vi "isForEditing.vi"(8 "error in (no error)":errorcluster, 11 "RampAction in":refnum<class "RampAction.lvclass">) -> (0 "error out":errorcluster, 2 "editing?":bool, 3 "RampAction out":refnum<class "RampAction.lvclass">)   [LabVIEW 2009, in "Views.lvlib" / "ScriptEditor.lvlib" / "RampAction.lvclass"]
uses:
  RampAction.lvclass
  Tools/Scripting/ScriptingEvent/ScriptEvents/Ramp/RampEvent/RampEvent.lvclass
  ActionPanel.lvclass
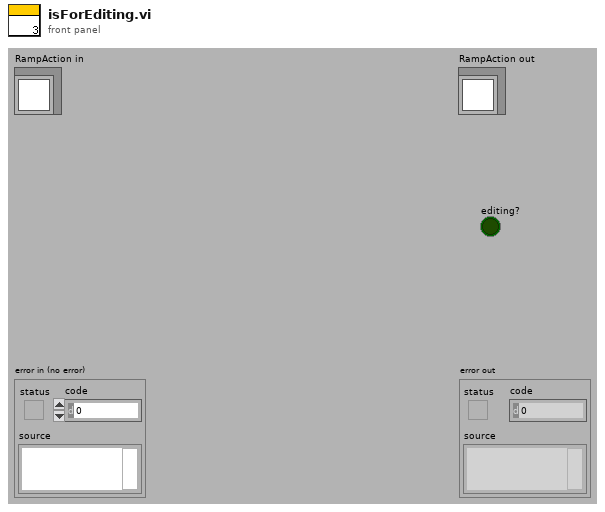
[diagram p1: front panel]
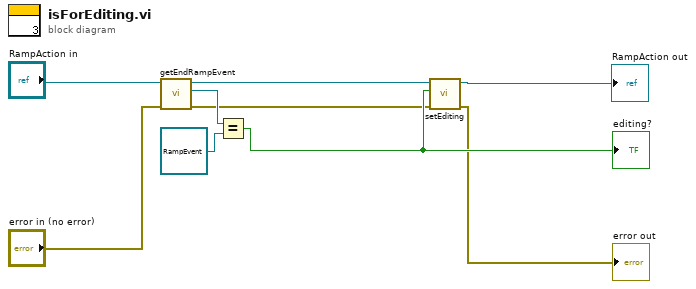
[diagram p0: block diagram]
diagram:
  n1 = call "getEndRampEvent.vi"("error in (no error)"="error in (no error)", "RampAction in"="RampAction in") -> ("error out"=w3:errorcluster, "EndScriptEvent"=w7:refnum<class "ScriptEvent.lvclass">, "RampAction out"=w5:refnum<class "RampAction.lvclass">)  [unwired: 7 in]
  n2 = Equal?(x=w7, y=refnum<class "RampEvent.lvclass"> refnum ("Tools.lvlib:Scripting.lvlib:RampEvent.lvclass")) -> (x = y?=w4:bool)
  "editing?" <- w4
  n3 = call "setEditing.vi"("error in (no error)"=w3, "editing?"=w4, "ActionPanel.lvclass in"=w5) -> ("error out"=→"error out":errorcluster, "ActionPanel.lvclass out"=→"RampAction out":refnum<class "RampAction.lvclass">)  [unwired: 7 in]
